vi "DataLengthBytes.vi"(10 "Is masked?":bool=TRUE, 11 "Data":u8[](array[numeric])) -> (3 "Length Bytes":u8[](array[numeric]))   [LabVIEW 2021, in "WebSockets.lvlib" / "WebSocket.lvclass"]
doc: "Generates the message length bytes of the WebSockets packet. A varying number of bytes is used to indicate the length of the data.\nWebSockets 2.0.1.40\nSam Sharp - MediaMongrels Ltd\nCopyright (c) 2019, MediaMongrels Ltd"
uses:
  WebSocket.lvclass
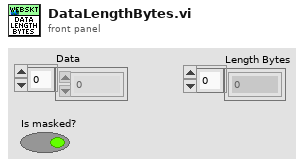
[diagram p1: front panel]
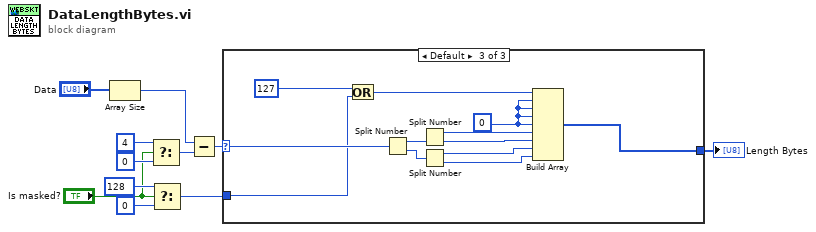
[diagram p0: block diagram]
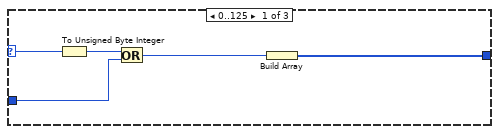
[diagram p2: hidden frame]
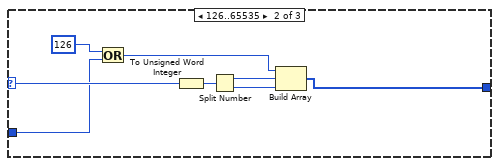
[diagram p3: hidden frame]
diagram:
  n1 = Array Size(array="Data") -> (size(s)=w1:i32)
  n2 = Select(t=4, s="Is masked?", f=0) -> (s? t:f=w4:i32)
  n3 = Select(t=u8 128, s="Is masked?", f=u8 0) -> (s? t:f=w9:u8)
  n4 = Subtract(x=w1, y=w4) -> (x-y=w8:i32)
  n5 = case shown="Default" w8 {
    selector: w8 -> [w13 w21 w29]
    tunnel: [w16 w20 w28] -> w3
    tunnel: w9 -> [w15 w17 w26]
    frame 0..125 {
      n6 = To Unsigned Byte Integer(number=w13) -> (unsigned 8bit integer=w14:u8)
      n7 = Or(x=w14, y=w15) -> (x .or. y?=w12:u8)
      n8 = Build Array(w12) -> (w16:u8[])
    }
    frame 126..65535 {
      n9 = Or(x=u8 126, y=w17) -> (x .or. y?=w18:u8)
      n10 = To Unsigned Word Integer(number=w21) -> (unsigned 16bit integer=w24:u16)
      n11 = Split Number(x=w24) -> (hi(x)=w23:u8, lo(x)=w22:u8)
      n12 = Build Array(w18, w23, w22) -> (w20:u8[])
    }
    frame Default {
      w30 = u8 0
      n13 = Or(x=u8 127, y=w26) -> (x .or. y?=w25:u8)
      n14 = Split Number(x=w29) -> (hi(x)=w36:u16, lo(x)=w35:u16)
      n15 = Split Number(x=w36) -> (hi(x)=w34:u8, lo(x)=w33:u8)
      n16 = Split Number(x=w35) -> (hi(x)=w32:u8, lo(x)=w31:u8)
      n17 = Build Array(w25, w30, w30, w30, w30, w34, w33, w32, w31) -> (w28:u8[])
    }
  }
  "Length Bytes" <- w3
